vi "Get Info Log.vi"(8 "error in (no error)":errorcluster, 10 "Parse All":bool, 11 "Plugin Manager in":refnum<class "CIFPluginManager.lvclass">) -> (0 "error out":errorcluster, 2 "Filtered Info Entries":string, 3 "Plugin Manager out":refnum<class "CIFPluginManager.lvclass">)   [LabVIEW 2021, in "CIFPluginManager.lvclass"]
uses:
  CIFPluginManager.lvclass
  CIFPluginManager.lvclass/CIFPluginManager.ctl
  <vilib>/CIF Foundation/CIF Core/CIFUtilities/CIFLogs/CIFLogs.lvlib
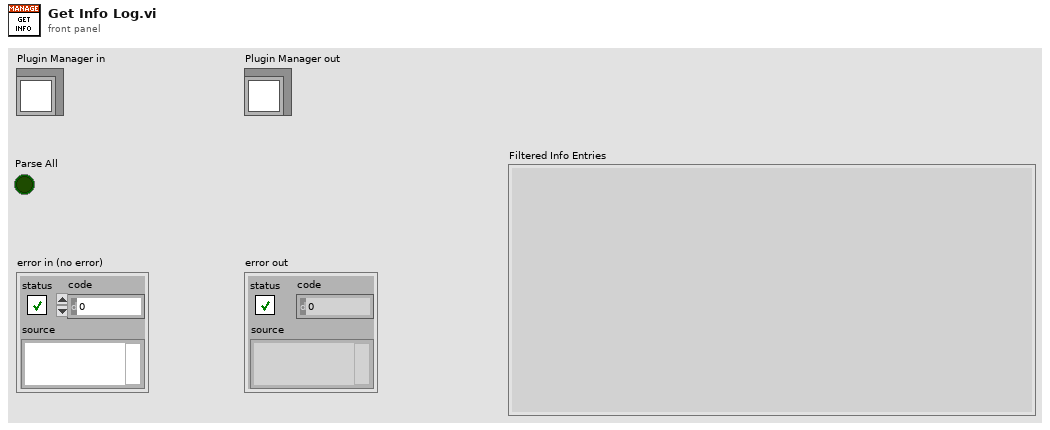
[diagram p1: front panel]
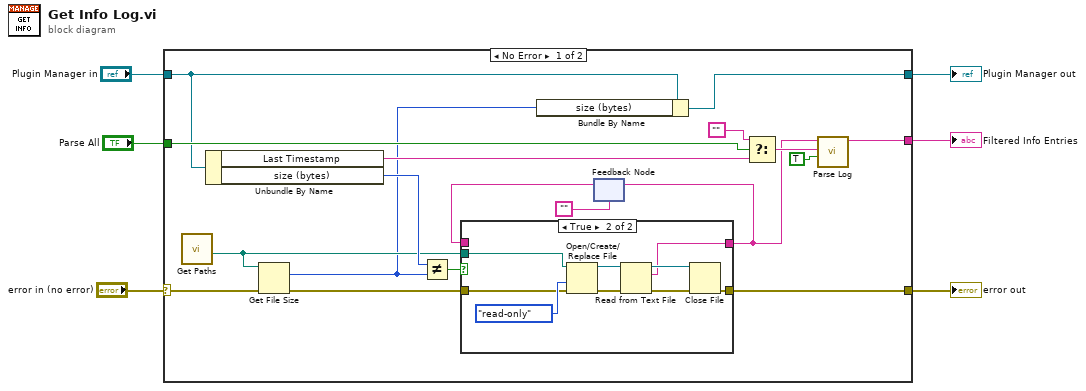
[diagram p0: block diagram]
diagram:
  n1 = case shown="No Error" "error in (no error)" {
    selector: "error in (no error)" -> [w18 w37]
    tunnel: [w24 w37] -> w1
    tunnel: [w8 w36] -> w3
    tunnel: "Plugin Manager in" -> [w9 w36]
    tunnel: [w21 _] -> w2
    tunnel: "Parse All" -> [w23 _]
    frame No Error {
      n2 = call <vilib>:"Get Paths.vi"() -> ("Info Log"=w11:path)  [unwired: 9 in, 2 out]
      n3 = Unbundle By Name(w9) -> ("Last Timestamp"=w10:string, "size (bytes)"=w16:i64)
      n4 = Get File Size(file=w11, error in=w18) -> (size (in bytes)=w7:i64, 0:w17:errorcluster)  [unwired: 1 out]
      n5 = Not Equal?(x=w16, y=w7) -> (x != y?=w15:bool)
      n6 = Bundle By Name(cluster=w9, "size (bytes)"=w7) -> (w8:refnum<class "CIFPluginManager.lvclass">)
      n7 = feedback #1("") -> (w12:string)
      n8 = case shown="True" w15 {
        tunnel: [w25 w31] -> w24
        tunnel: w11 -> [_ w29]
        tunnel: w17 -> [w25 w28]
        tunnel: [w26 w27] -> w14
        tunnel: w12 -> [w26 _]
        frame False {
        }
        frame True {
          n9 = Open/Create/Replace File(file path (use dialog)=w29, error in=w28, access (0:read/write)=enum16{"read/write", "read-only", "write-only"}."read-only") -> (refnum out=w34:refnum<file>, error out=w33:errorcluster)  [unwired: 3 in, 1 out]
          n10 = Read from Text File(file (use dialog)=w34, error in=w33) -> (refnum out=w35:refnum<file>, text=w27:string, error out=w32:errorcluster)  [unwired: 2 in, 1 out]
          n11 = Close File(refnum=w35, error in=w32) -> (error out=w31:errorcluster)  [unwired: 1 out]
        }
      }
      n12 = feedback-in #1(w14) -> ()
      n13 = Select(t="", s=w23, f=w10) -> (s? t:f=w22:string)
      n14 = call <vilib>:"Parse Log.vi"("Strip Timestamp"=TRUE, "Index Timestamp"=w22, "Log"=w14) -> ("Filtered Config Entries"=w21:string)  [unwired: 8 in]
    }
    frame Error {
    }
  }
  "error out" <- w1
  "Plugin Manager out" <- w3
  "Filtered Info Entries" <- w2
